vi "GPS Loop.vi"() -> (0 "VI Refnum":refnum<vi>)   [LabVIEW 2012]
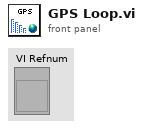
[diagram p1: front panel]
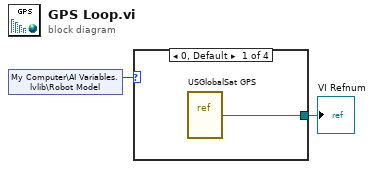
[diagram p0: block diagram]
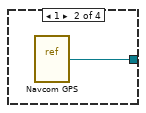
[diagram p2: hidden frame]
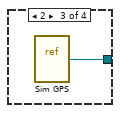
[diagram p3: hidden frame]
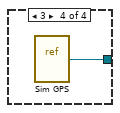
[diagram p4: hidden frame]
diagram:
  n1 = shared-variable "My Computer\\AI Variables.lvlib\\Robot Model"() -> (w2:u16)  [unwired: 1 in, 1 out]
  n2 = case shown="0, Default" w2 {
    tunnel: [w3 w4 w5 w6] -> w1
    frame 0, Default {
      n3 = vi-ref "USGlobalSat GPS.vi"() -> (w3:refnum<vi>)
    }
    frame 1 {
      n4 = vi-ref "Navcom GPS.vi"() -> (w4:refnum<vi>)
    }
    frame 2 {
      n5 = vi-ref "Sim GPS.vi"() -> (w5:refnum<vi>)
    }
    frame 3 {
      n6 = vi-ref "Sim GPS.vi"() -> (w6:refnum<vi>)
    }
  }
  "VI Refnum" <- w1
